vi "TSPopup.Register.vi"(4 "Col (unwired = all columns)":i32=-2, 6 "Row (unwired = all rows)":i32=-2, 7 "Tag (none)":string, 8 "error in (no error)":errorcluster, 9 "Parameters":T1={"Prop Type"=enum."String", "Initial Value"=variant, "Caption Strings"=[], "Ring Strings"=[], "Cell Rect"={"left"=0, "top"=0, "right"=0, "bottom"=0}, "Mouse Coords"={"x"=0, "y"=0}, "Call Data"=variant}, 10 "Ctl Refnum":refnum<vi>, 11 "TSPopup in":refnum<class "TSPopup.lvclass">) -> (0 "error out":errorcluster, 2 "dup ref out":refnum<vi>, 3 "TSPopup out":refnum<class "TSPopup.lvclass">)   [LabVIEW 2016, in "TSPopup.lvlib" / "TSPopup.lvclass"]
doc: "Register a control location with some associated Popup Parameters. These will be retrieved by using the \"TSPopup.Lookup.vi\" in a <Mouse Down?> event. \n\nRegistration can be done for an exact cell, a column, a row, or an entire control. Retrieval of parameters will be done by searching in that order.\n\n<B>Ctl Refnum</B> - Refnum of control that is being registered (allowed control types : String, Table, Listbox, Multicolumn Listbox, Tree)\n<B>Popup Parameters</B> - Parameters for showing the Type Sensitive Popup.\n<B>Tag</B> - For tree controls, this is the row's tag. Unwired or blank equals all rows.\n<B>Row</B> - Row being registered. Unwired or (< -1) equals all rows.\n<B>Col</B> - Column being registered. Unwired or (< -1) equals all rows.\n\nType Sensitive Popup \nCopyright © 2007, J. David Saunders\nAll rights reserved."
uses:
  <userlib>/TSPopup/TSPopup.lvclass
  <userlib>/TSPopup/TSPopup.Popup Call Parameters.ctl
  <userlib>/TSPopup/TSPopup.Data Type.ctl
  <userlib>/TSPopup/TSPopup.lvclass/TSPopup.ctl
panel:
  # "Type Sensitive Popup \nCopyright © 2007, J. David Saunders\nAll rights reserved."
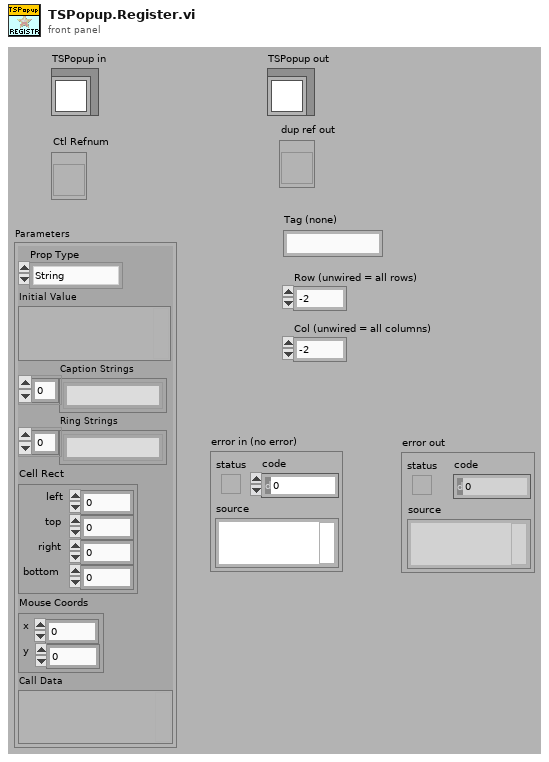
[diagram p1: front panel]
types:
  T1 = typedef "TSPopup.lvlib/TSPopup.lvclass/TSPopup.Popup Call Parameters.ctl" = cluster{"Prop Type":T2, "Initial Value":variant, "Caption Strings":string[], "Ring Strings":string[], "Cell Rect":cluster{"left":i16, "top":i16, "right":i16, "bottom":i16}, "Mouse Coords":cluster{"x":i16, "y":i16}, "Call Data":variant}
  T2 = typedef "TSPopup.lvlib/TSPopup.lvclass/TSPopup.Data Type.ctl" = enum16{"Unkown", "NO POPUP", "String", "Integer", "Float", "Color", "Boolean", "Ring", "Captioned String", "Captioned Integer", "Button Color", "2 Int Cluster", "4 Int Cluster", "check"}
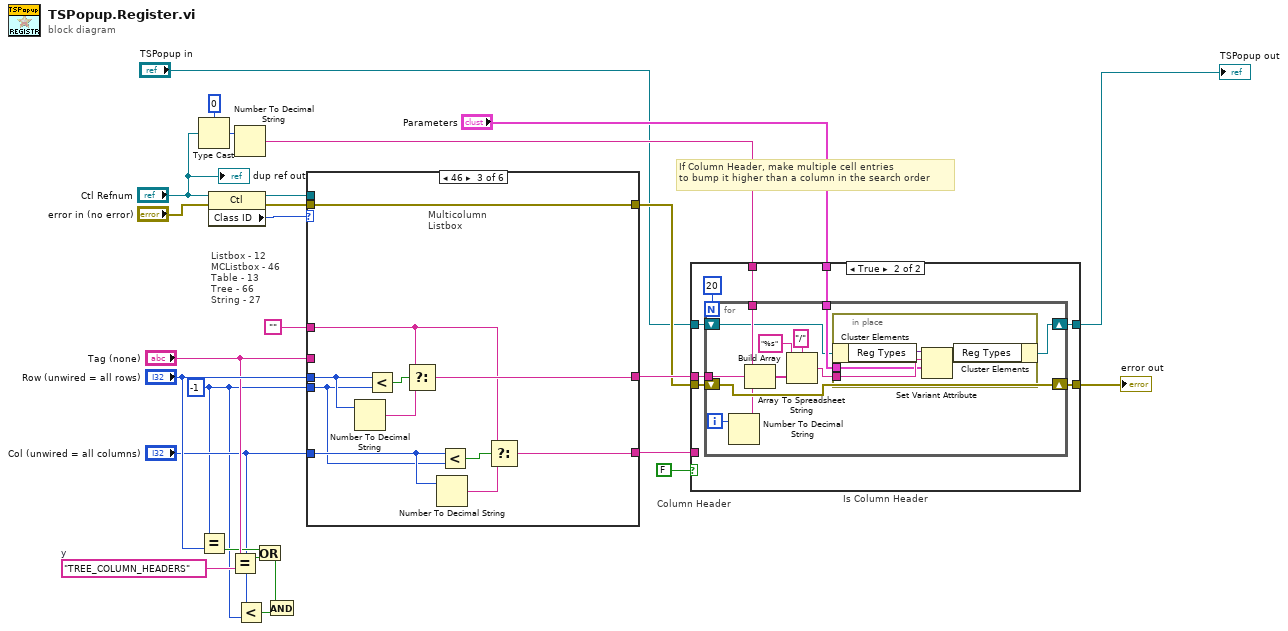
[diagram p0: block diagram]
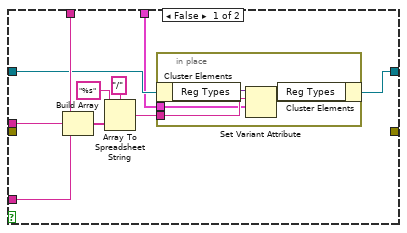
[diagram p2: hidden frame]
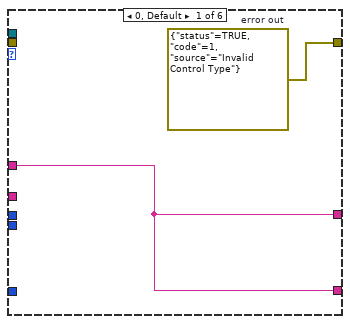
[diagram p3: hidden frame]
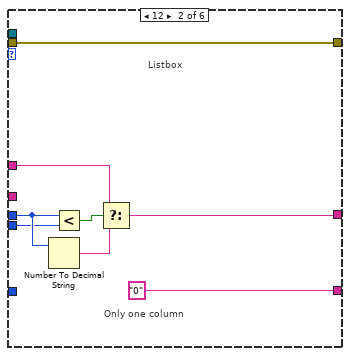
[diagram p4: hidden frame]
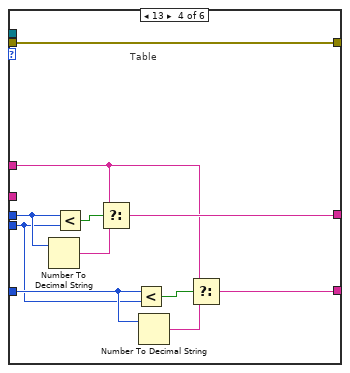
[diagram p5: hidden frame]
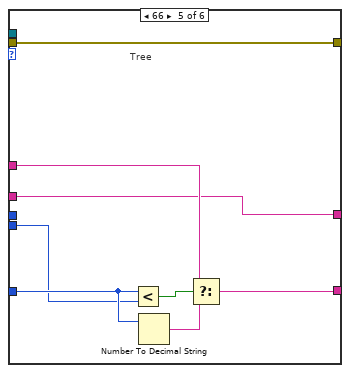
[diagram p6: hidden frame]
diagram:
  w13 = "TREE_COLUMN_HEADERS"  # y
  w6 = -1 ("y")
  # "If Column Header, make multiple cell entries\nto bump it higher than a column in the search order"
  # "Column Header"
  # "Listbox - 12\nMCListbox - 46\nTable - 13\nTree - 66\nString - 27"
  n1 = Type Cast(type=0, x="Ctl Refnum") -> (*(type *) &x=w23:i32)
  n2 = Equal?(x=w6, y="Row (unwired = all rows)") -> (x = y?=w11:bool)
  n3 = property class="Ctl"(reference="Ctl Refnum", error in="error in (no error)") -> (reference out=w25:refnum<vi>, error out=w17:errorcluster, "Class ID"=w26:u32)
  n4 = Equal?(x="Tag (none)", y=w13) -> (x = y?=w12:bool)
  n5 = Number To Decimal String(number=w23) -> (decimal integer string=w22:string)  [unwired: 1 in]
  n6 = Less?(x="Col (unwired = all columns)", y=w6) -> (x < y?=w5:bool)
  n7 = Or(x=w11, y=w12) -> (x .or. y?=w4:bool)
  n8 = And(x=w4, y=w5) -> ()  [unwired: 1 out]
  n9 = case shown="46" w26 {
    tunnel: w25 -> [_ _ _ _ _ _]
    tunnel: "Tag (none)" -> [_ _ _ _ w63 _]
    tunnel: "Row (unwired = all rows)" -> [_ w31 w40 w52 _ _]
    tunnel: "Col (unwired = all columns)" -> [_ _ w39 w50 w61 _]
    tunnel: "" -> [w28 w35 w43 w54 w64 w68]
    tunnel: [w28 w34 w46 w57 w63 w68] -> w20
    tunnel: [w28 "0" w44 w55 w65 w68] -> w19
    tunnel: w17 -> [_ w32 w42 w53 w62 w67]
    tunnel: [w27 w32 w42 w53 w62 w67] -> w8
    tunnel: w6 -> [_ w30 w37 w49 w60 _]
    frame 0, Default {
      w27 = errorcluster {"status"=TRUE, "code"=1, "source"="Invalid Control Type"}  # error out
    }
    frame 12 {
      # "Only one column"
      # "Listbox"
      n10 = Number To Decimal String(number=w31) -> (decimal integer string=w36:string)  [unwired: 1 in]
      n11 = Less?(x=w31, y=w30) -> (x < y?=w29:bool)
      n12 = Select(t=w35, s=w29, f=w36) -> (s? t:f=w34:string)
    }
    frame 46 {
      # "Multicolumn\nListbox"
      n13 = Number To Decimal String(number=w40) -> (decimal integer string=w47:string)  [unwired: 1 in]
      n14 = Less?(x=w40, y=w37) -> (x < y?=w41:bool)
      n15 = Select(t=w43, s=w41, f=w47) -> (s? t:f=w46:string)
      n16 = Number To Decimal String(number=w39) -> (decimal integer string=w45:string)  [unwired: 1 in]
      n17 = Less?(x=w39, y=w37) -> (x < y?=w38:bool)
      n18 = Select(t=w43, s=w38, f=w45) -> (s? t:f=w44:string)
    }
    frame 13 {
      # "Table"
      n19 = Number To Decimal String(number=w52) -> (decimal integer string=w58:string)  [unwired: 1 in]
      n20 = Less?(x=w52, y=w49) -> (x < y?=w51:bool)
      n21 = Select(t=w54, s=w51, f=w58) -> (s? t:f=w57:string)
      n22 = Less?(x=w50, y=w49) -> (x < y?=w48:bool)
      n23 = Number To Decimal String(number=w50) -> (decimal integer string=w56:string)  [unwired: 1 in]
      n24 = Select(t=w54, s=w48, f=w56) -> (s? t:f=w55:string)
    }
    frame 66 {
      # "Tree"
      n25 = Less?(x=w61, y=w60) -> (x < y?=w59:bool)
      n26 = Number To Decimal String(number=w61) -> (decimal integer string=w66:string)  [unwired: 1 in]
      n27 = Select(t=w64, s=w59, f=w66) -> (s? t:f=w65:string)
    }
    frame 27 {
      # "String"
    }
  }
  n28 = case "Is Column Header" shown="True" FALSE {
    tunnel: w22 -> [w75 w90]
    tunnel: w20 -> [w74 w89]
    tunnel: w19 -> [w73 _]
    tunnel: [_ w88] -> w10
    tunnel: "Parameters" -> [w69 w87]
    tunnel: w8 -> [_ w86]
    tunnel: "TSPopup in" -> [w72 w84]
    tunnel: [w71 w83] -> w1
    frame False {
      n29 = Build Array(w75, w74, w73) -> (w78:string[])
      n30 = Array To Spreadsheet String(delimiter (Tab)="/", array=w78, 3:"%s" ("format string")) -> (spreadsheet string=w70:string)
      n31 = in-place {
        in-place-border: w70 -> [w80]
        in-place-border: w69 -> [w79]
        n32 = in-place-cluster #1(w72) -> ("Reg Types"=w82:variant)
        n33 = Set Variant Attribute(Variant=w82, name=w80, value=w79) -> (Variant out=w81:variant)  [unwired: 1 in, 2 out]
        n34 = in-place-cluster #1("Reg Types"=w81) -> (w71:refnum<class "TSPopup.lvclass">)
      }
    }
    frame True {
      n35 = for {
        N: 20 -> [_]
        tunnel: w90 -> [w99]
        tunnel: w89 -> [w98]
        tunnel: w87 -> [w93]
        shift-right: [w97] -> w88
        shift-left: w86 -> [w97]
        shift-right: [w91] -> w83
        shift-left: w84 -> [w92]
        i -> [w96]
        n36 = Number To Decimal String(number=w96) -> (decimal integer string=w95:string)  [unwired: 1 in]
        n37 = Build Array(w99, w98, w95) -> (w102:string[])
        n38 = Array To Spreadsheet String(delimiter (Tab)="/", array=w102, 3:"%s" ("format string")) -> (spreadsheet string=w94:string)
        n39 = in-place {
          in-place-border: w94 -> [w104]
          in-place-border: w93 -> [w103]
          n40 = in-place-cluster #2(w92) -> ("Reg Types"=w106:variant)
          n41 = Set Variant Attribute(Variant=w106, name=w104, value=w103) -> (Variant out=w105:variant)  [unwired: 1 in, 2 out]
          n42 = in-place-cluster #2("Reg Types"=w105) -> (w91:refnum<class "TSPopup.lvclass">)
        }
      }
    }
  }
  "error out" <- w10
  "TSPopup out" <- w1
  "dup ref out" <- "Ctl Refnum"
